vi "Allocate memory.vi"(8 "nob":u32=4, 9 "nos":u32=1100, 11 "Camera error in":errorcluster) -> (3 "Camera error out":errorcluster)   [LabVIEW 2018]
uses:
  board.vis/Globals.vi
  Stresing_dual_cam.lvclass
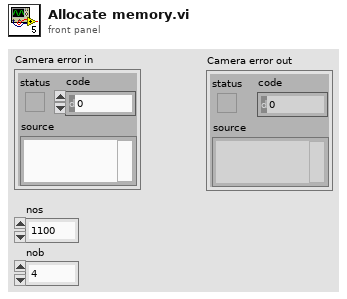
[diagram p1: front panel]
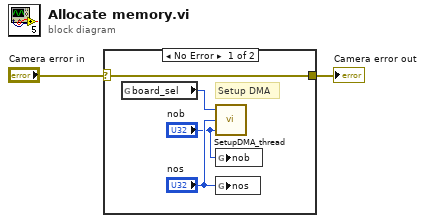
[diagram p0: block diagram]
diagram:
  n1 = case shown="No Error" "Camera error in" {
    selector: "Camera error in" -> [w3 w7]
    tunnel: [w3 w7] -> w1
    frame No Error {
      # "Setup DMA"
      n2 = global read "Globals.vi" "board_sel"() -> (w6:u32)
      n3 = call "SetupDMA_thread.vi"("blocks"="nob", "nos"="nos", "Board_sel"=w6) -> ()  [unwired: 2 in]
      n4 = global write "Globals.vi" "nob"("nob") -> ()
      n5 = global write "Globals.vi" "nos"("nos") -> ()
    }
    frame Error {
    }
  }
  "Camera error out" <- w1
